vi "Enqueue N States.vi"(0 "Queue Ref In":refnum<queue>, 5 "N States":string, 11 "error in (no error)":errorcluster) -> (4 "Queue Ref Out":refnum<queue>, 15 "error out":errorcluster)   [LabVIEW 2019, in "Queue Driver.lvlib"]
uses:
  Queue Driver.lvlib
  TypeDefs/Queue Data.ctl
  TypeDefs/Queue Operation.ctl
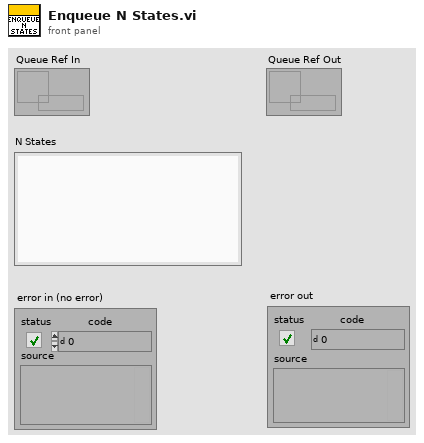
[diagram p1: front panel]
types:
  T1 = typedef "Queue Driver.lvlib/Queue Operation.ctl" = enum16{"Create", "Enqueue", "EnqueueN", "Dequeue", "Flush", "Destroy"}
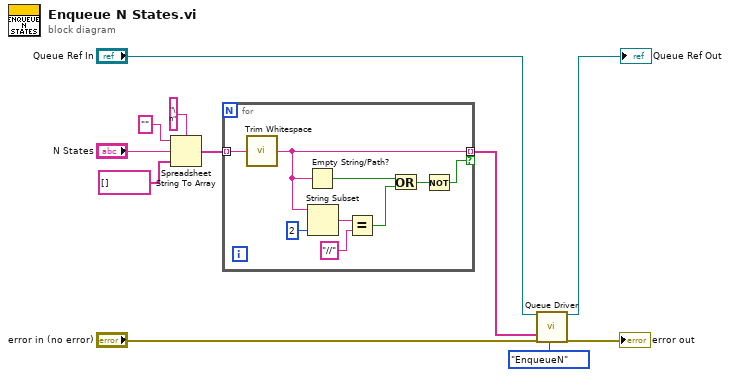
[diagram p0: block diagram]
diagram:
  n1 = Spreadsheet String To Array(delimiter (Tab)="\n", format string="", spreadsheet string="N States", array type (2D Dbl)=string[] [] ("N States")) -> (array=w2:string[])
  n2 = for {
    tunnel: w2 -> [w20] mode=indexing
    tunnel: [w16] -> w1 mode=indexing if=w12
    n3 = call <vilib>:"Trim Whitespace.vi"("string"=w20) -> ("trimmed string"=w16:string)  [unwired: 1 in]
    n4 = Empty String/Path?(string/path=w16) -> (empty?=w15:bool)
    n5 = String Subset(string=w16, length (rest)=2 ("length (rest)")) -> (substring=w18:string)  [unwired: 1 in]
    n6 = Equal?(x=w18, y="//") -> (x = y?=w14:bool)
    n7 = Or(x=w15, y=w14) -> (x .or. y?=w13:bool)
    n8 = Not(x=w13) -> (.not. x?=w12:bool)
  }
  n9 = call "Queue Driver.vi"("Queue Ref In"="Queue Ref In", "EnqueueN States"=w1, "error in (no error)"="error in (no error)", "Queue Operation"=Queue_Operation."EnqueueN") -> ("Queue Ref Out"=→"Queue Ref Out":refnum<queue>, "error out"=→"error out":errorcluster)  [unwired: 12 in, 2 out]
